vi "rqcAlice Modulator (FPGA).vi"(0 "pulse arrived":bool, 2 "reset":bool, 7 "DAC random value":u32, 9 "rqcAlice PM.config":T1) -> (4 "DAC level":u8, 6 "DAC value":u16, 10 "DAC value changed":bool=TRUE)   [LabVIEW 2018]
uses:
  Custom Controls/Phase Modulator/rqcAlice Mod.Config.ctl
  <vilib>/RQC/FPGA Basic Logic/Counters/Counter (U8).vi
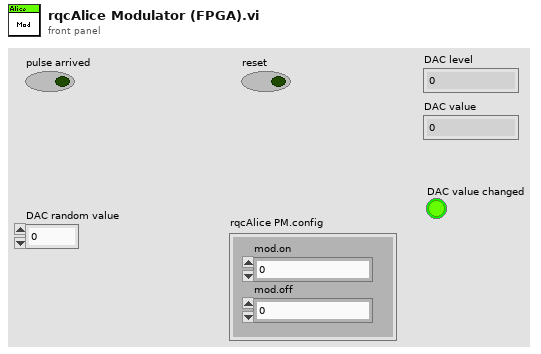
[diagram p1: front panel]
types:
  T1 = typedef "rqcAlice Mod.Config.ctl" = cluster{"mod.on":u8, "mod.off":u8}
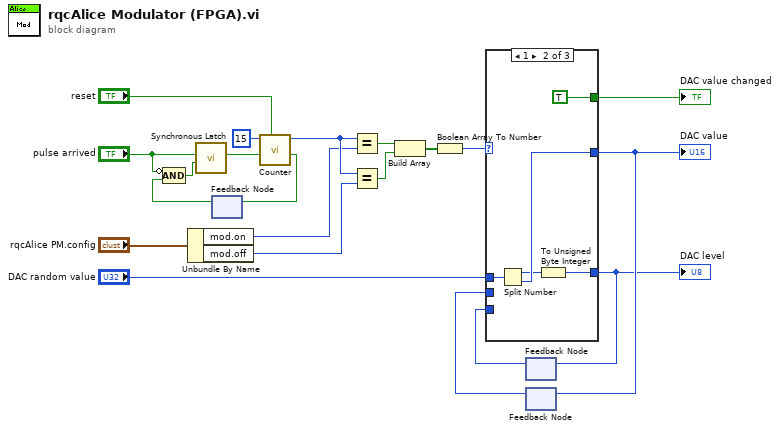
[diagram p0: block diagram]
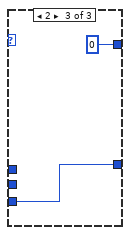
[diagram p3: hidden frame]
diagram:
  n1 = Unbundle By Name("rqcAlice PM.config") -> ("mod.on"=w11:u8, "mod.off"=w10:u8)
  n2 = feedback #1() -> (w17:bool)  [unwired: 1 in]
  n3 = Compound Arithmetic op=AND(invert "pulse arrived", w17) -> (w19:bool)
  n4 = call <vilib>:"Synchronous Latch.vi"("clear"=w19, "set"="pulse arrived") -> ("out"=w20:bool)  [unwired: 9 in]
  n5 = call-poly <vilib>:"Counter.vi"("reset"="reset", "increment"=w20, "bound"=u8 15) -> ("done"=w18:bool, "count out"=w16:u8)  [unwired: 7 in]
  n6 = feedback-in #1(w18) -> ()
  n7 = Equal?(x=w16, y=w11) -> (x = y?=w5:bool)
  n8 = Equal?(x=w16, y=w10) -> (x = y?=w15:bool)
  n9 = Build Array(w5, w15) -> (w13:bool[])
  n10 = Boolean Array To Number(Boolean array=w13) -> (number=w14:u8)
  n11 = feedback #2() -> (w6:u8)  [unwired: 1 in]
  n12 = feedback #3() -> (w8:u16)  [unwired: 1 in]
  n13 = case shown="1" w14 {
    tunnel: [w23 w25 u16 0 ("DAC value")] -> w9
    tunnel: w8 -> [w23 _ _]
    tunnel: [w22 w28 w29] -> w7
    tunnel: w6 -> [w22 _ w29]
    tunnel: [_ TRUE _] -> w4
    tunnel: "DAC random value" -> [_ w26 _]
    frame 0, Default {
    }
    frame 1 {
      n14 = Split Number(x=w26) -> (hi(x)=w24:u16, lo(x)=w25:u16)
      n15 = To Unsigned Byte Integer(number=w24) -> (unsigned 8bit integer=w28:u8)
    }
    frame 2 {
    }
  }
  "DAC value" <- w9
  "DAC level" <- w7
  "DAC value changed" <- w4
  n16 = feedback-in #2(w7) -> ()
  n17 = feedback-in #3(w9) -> ()
